vi "Sending String CMD Data and Password.vi"(0 "TCP Ref In":refnum<k5>, 1 "Time Out(ms)":i32=100, 5 "CMD In":string, 7 "Data  In":string, 9 "Password":string, 11 "error in (no error)":errorcluster) -> (4 "TCP Ref Out":refnum<k5>, 15 "error out":errorcluster)   [LabVIEW 2024]
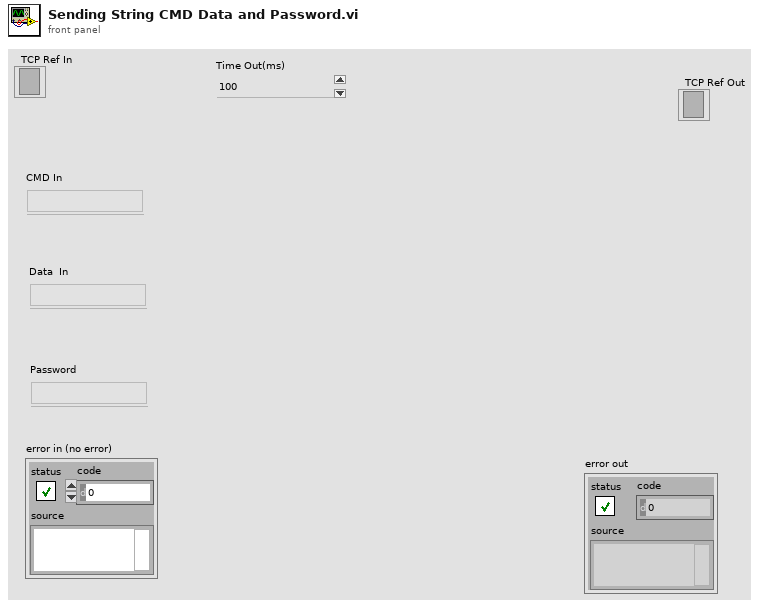
[diagram p1: front panel]
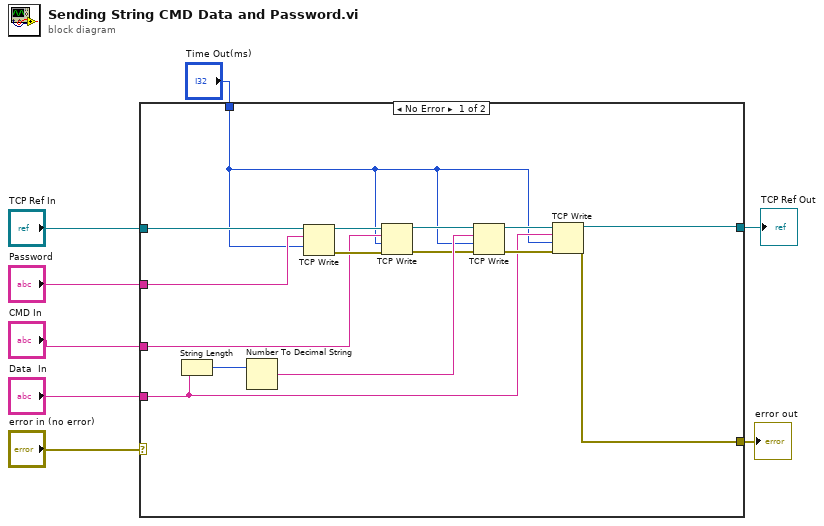
[diagram p0: block diagram]
diagram:
  n1 = case shown="No Error" "error in (no error)" {
    selector: "error in (no error)" -> [_ w25]
    tunnel: [w9 w25] -> w7
    tunnel: "Time Out(ms)" -> [w11 _]
    tunnel: "TCP Ref In" -> [w21 w24]
    tunnel: [w10 w24] -> w4
    tunnel: "Password" -> [w20 _]
    tunnel: "CMD In" -> [w19 _]
    tunnel: "Data  In" -> [w12 _]
    frame No Error {
      n2 = String Length(string=w12) -> (length=w17:i32)
      n3 = Number To Decimal String(number=w17) -> (decimal integer string=w16:string)  [unwired: 1 in]
      n4 = TCP Write(connection ID=w21, data in=w20, 9:w11) -> (connection ID out=w23:refnum<k5>, error out=w22:errorcluster)  [unwired: 1 in, 1 out]
      n5 = TCP Write(connection ID=w23, data in=w19, error in (no error)=w22, 9:w11) -> (connection ID out=w18:refnum<k5>, error out=w15:errorcluster)  [unwired: 1 out]
      n6 = TCP Write(connection ID=w18, data in=w16, error in (no error)=w15, 9:w11) -> (connection ID out=w14:refnum<k5>, error out=w13:errorcluster)  [unwired: 1 out]
      n7 = TCP Write(connection ID=w14, data in=w12, error in (no error)=w13, 9:w11) -> (connection ID out=w10:refnum<k5>, error out=w9:errorcluster)  [unwired: 1 out]
    }
    frame Error {
    }
  }
  "error out" <- w7
  "TCP Ref Out" <- w4
